vi "Is Point In Shape.vi"(8 "error in (no error)":errorcluster, 10 "Point":cluster{"Horizontal":i32, "Vertical":i32}, 11 "Triangle in":refnum<class "Triangle.lvclass">) -> (0 "error out":errorcluster, 2 "Point In Shape?":bool, 3 "Triangle out":refnum<class "Triangle.lvclass">)   [LabVIEW 2015, in "Triangle.lvclass"]
uses:
  Triangle.lvclass
  <vilib>/Analysis/geometry.llb/Point in Polygon Position.ctl
  Interfaces/Shape/Shape.lvclass/Shape.ctl
  <vilib>/Analysis/geometry.llb/Point in Polygon (Scalar).vi
  Interfaces/Shape/Shape.lvclass
  <vilib>/Analysis/NI_AAL_Geometry.lvlib
panel:
  # "NOTICE -- YOU MUST LEAVE THIS NOTICE IN PLACE.\n\nCopyright (c) 2017, LIANG LIU Shawn.Liu.cn@gmail.com\nAll rights reserved.\n\nRedistribution and use in source and binary forms, with or without modification, are permitted provided that the following conditions are met:\n-Redistributions of source code must retain the above copyright notice, this list of conditions and the following disclaimer.\n-Redistributions in binary form must reproduce the above copyright notice, this list of conditions and the following disclaimer in the documentation and/or other materials provided with the distribution.\n-Neither the name of the eLp nor the names of its contributors may be used to endorse or promote products derived from this software without specific prior written permission.\n\nTHIS SOFTWARE IS PROVIDED BY THE COPYRIGHT HOLDERS AND CONTRIBUTORS \"AS IS\" AND ANY EXPRESS OR IMPLIED WARRANTIES, INCLUDING, BUT NOT LIMITED TO, THE IMPLIED WARRANTIES OF MERCHANTABILITY AND FITNESS FOR A PARTICULAR PURPOSE ARE DISCLAIMED. IN NO EVENT SHALL THE COPYRIGHT HOLDER OR CONTRIBUTORS BE LIABLE FOR ANY DIRECT, INDIRECT, INCIDENTAL, SPECIAL, EXEMPLARY, OR CONSEQUENTIAL DAMAGES (INCLUDING, BUT NOT LIMITED TO, PROCUREMENT OF SUBSTITUTE GOODS OR SERVICES; LOSS OF USE, DATA, OR PROFITS; OR BUSINESS INTERRUPTION) HOWEVER CAUSED AND ON ANY THEORY OF LIABILITY, WHETHER IN CONTRACT, STRICT LIABILITY, OR TORT (INCLUDING NEGLIGENCE OR OTHERWISE) ARISING IN ANY WAY OUT OF THE USE OF THIS SOFTWARE, EVEN IF ADVISED OF THE POSSIBILITY OF SUCH DAMAGE."
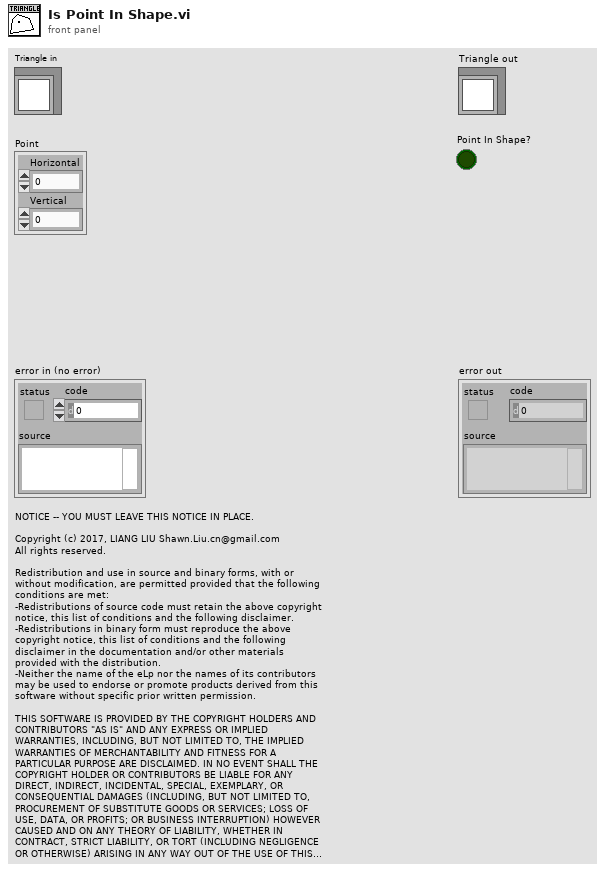
[diagram p1: front panel]
types:
  T1 = typedef "NI_AAL_Geometry.lvlib/Point in Polygon Position.ctl" = u16
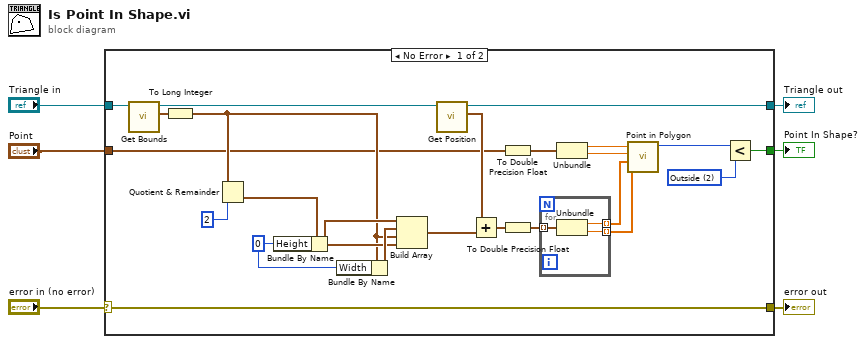
[diagram p0: block diagram]
diagram:
  n1 = case shown="No Error" "error in (no error)" {
    selector: "error in (no error)" -> [w7 w35]
    tunnel: "Triangle in" -> [w30 w34]
    tunnel: [w18 w34] -> w5
    tunnel: "Point" -> [w11 _]
    tunnel: [w9 _] -> w3
    tunnel: [w7 w35] -> w1
    frame No Error {
      w8 = T1 2 items=["Inside", "On Boundary", "Outside"] ("y")
      w26 = 0 ("Height")
      n2 = call "Get Bounds.vi"("Shape in"=w30) -> ("Bounds"=w21:cluster{"Width":u32, "Height":u32}, "Shape out"=w29:refnum<class "Triangle.lvclass">)  [unwired: 9 in]
      n3 = To Long Integer(number=w21) -> (32bit integer=w20:cluster{"Width":i32, "Height":i32})
      n4 = Quotient & Remainder(x=w20, y=2) -> (floor(x/y)=w28:cluster{"Width":i32, "Height":i32})  [unwired: 1 out]
      n5 = Bundle By Name(cluster=w28, "Height"=w26) -> (w24:cluster{"Width":i32, "Height":i32})
      n6 = Bundle By Name(cluster=w20, "Width"=w26) -> (w25:cluster{"Width":i32, "Height":i32})
      n7 = Build Array(w24, w25, w20, w24) -> (w23:cluster{"Width":i32, "Height":i32}[])
      n8 = call "Get Position.vi"("Shape in"=w29) -> ("Position"=w22:cluster{"Left":i32, "Top":i32}, "Shape out"=w18:refnum<class "Triangle.lvclass">)  [unwired: 9 in]
      n9 = Add(x=w22, y=w23) -> (x+y=w17:cluster{i32, i32}[])
      n10 = To Double Precision Float(number=w11) -> (double precision float=w10:cluster{"Horizontal":dbl, "Vertical":dbl})
      n11 = To Double Precision Float(number=w17) -> (double precision float=w16:cluster{dbl, dbl}[])
      n12 = for {
        tunnel: w16 -> [w33] mode=indexing
        tunnel: [w32] -> w15 mode=indexing
        tunnel: [w31] -> w14 mode=indexing
        n13 = Unbundle(w33) -> (w32:dbl, w31:dbl)
      }
      n14 = Unbundle(w10) -> ("Horizontal"=w13:dbl, "Vertical"=w12:dbl)
      n15 = call-poly <vilib>:"Point in Polygon.vi"("Polygon Y"=w14, "Polygon X"=w15, "y"=w12, "x"=w13) -> ("position"=w19:T1)  [unwired: 6 in, 1 out]
      n16 = Less?(x=w19, y=w8) -> (x < y?=w9:bool)
    }
    frame Error {
    }
  }
  "error out" <- w1
  "Triangle out" <- w5
  "Point In Shape?" <- w3
